vi "Running Average.vi"(8 "Error In":errorcluster, 11 "Async State Vars 2":T1) -> (0 "Error Out":errorcluster, 3 "Async State Vars out":T1)   [LabVIEW 2014, in "Waveform-Processing-Custom-Device Shared.lvlib" / "Running Average.lvlib"]
uses:
  Shared/Running Average/Running Average.lvlib
  Types/Async State Vars.ctl
  Types/Async FIFOs.ctl
  <vilib>/NI Veristand/Custom Device Waveform API/Single Waveform Read (DBL)/Single Waveform Read (DBL).lvclass
  <vilib>/NI Veristand/Custom Device Waveform API/Single Waveform Write (DBL)/Single Waveform Write (DBL).lvclass
  <vilib>/NI Veristand/Custom Device API/Waveform Data Reference.ctl
  <userlib>/Circular Buffer/Controls/Circular Buffer Operations.ctl
  <vilib>/Analysis/baseanly.llb/Mean (DBL).vi
  <userlib>/Circular Buffer/Instance VIs/Circular Buffer(2D DBL).vi
  <userlib>/Circular Buffer/Circular Buffer.lvlib
  <vilib>/Analysis/NI_AALBase.lvlib
  Waveform-Processing-Custom-Device Engine.lvlib
  <vilib>/NI Veristand/Custom Device API/Custom Device API.lvlib
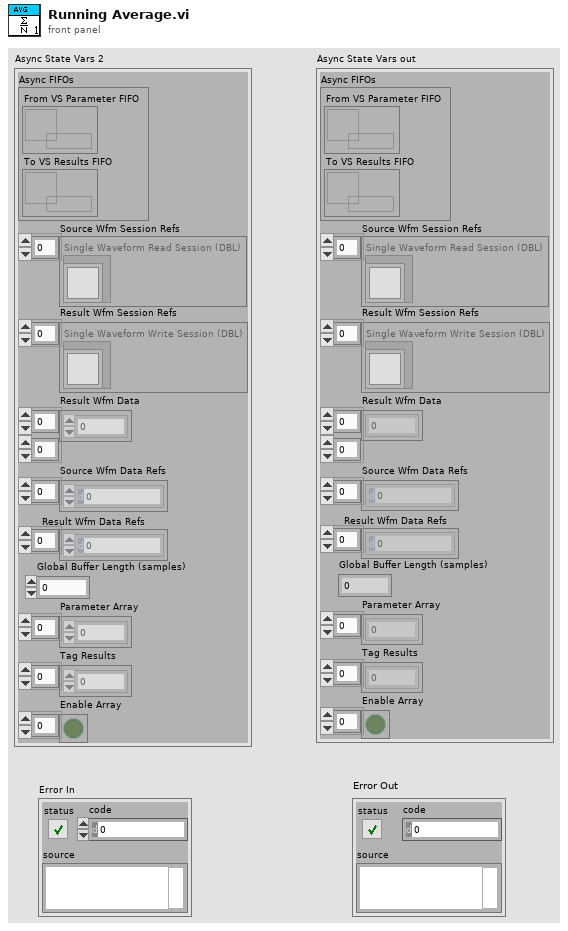
[diagram p1: front panel]
types:
  T1 = typedef "Waveform-Processing-Custom-Device Engine.lvlib/Async State Vars.ctl" = cluster{"Async FIFOs":T2, "Source Wfm Session Refs":refnum<class "Single Waveform Read (DBL).lvclass">[], "Result Wfm Session Refs":refnum<class "Single Waveform Write (DBL).lvclass">[], "Result Wfm Data":dbl[][], "Source Wfm Data Refs":T3[], "Result Wfm Data Refs":T3[], "Global Buffer Length (samples)":dbl, "Parameter Array":dbl[], "Tag Results":dbl[], "Enable Array":bool[]}
  T2 = typedef "Waveform-Processing-Custom-Device Engine.lvlib/Async FIFOs.ctl" = cluster{"From VS Parameter FIFO":refnum<k33>, "To VS Results FIFO":refnum<k33>}
  T3 = typedef "Custom Device API.lvlib/Waveform Data Reference.ctl" = i32
  T4 = typedef "Circular Buffer.lvlib/Circular Buffer Operations.ctl" = enum16{"Initialize", "Get Backlog", "Write", "Read (continuous)", "Read (most recent)"}
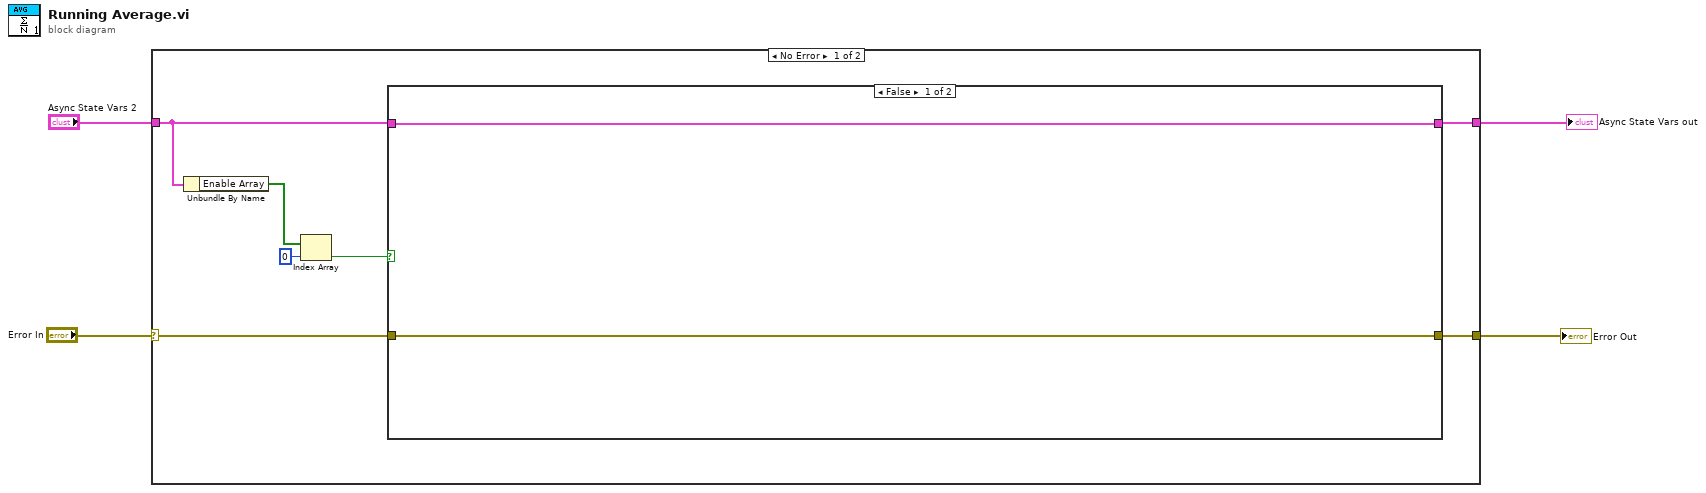
[diagram p0: block diagram]
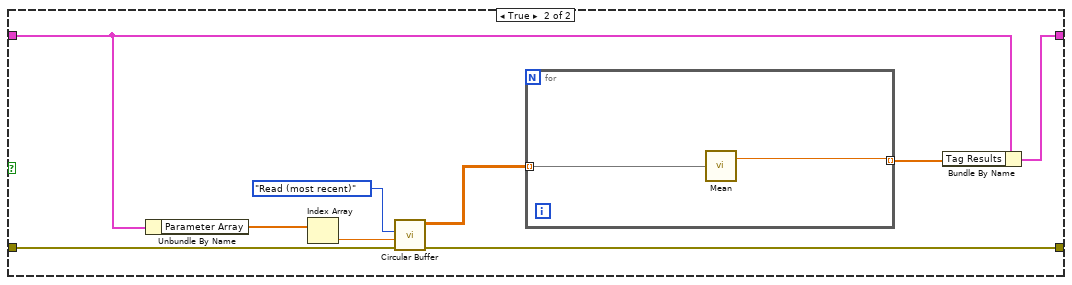
[diagram p2: hidden frame]
diagram:
  n1 = case shown="No Error" "Error In" {
    selector: "Error In" -> [w11 w26]
    tunnel: [w10 w26] -> w3
    tunnel: "Async State Vars 2" -> [w8 w25]
    tunnel: [w9 w25] -> w1
    frame No Error {
      n2 = Unbundle By Name(w8) -> ("Enable Array"=w7:bool[])
      n3 = Index Array(array=w7, index=0) -> (element=w6:bool)
      n4 = case shown="False" w6 {
        tunnel: w11 -> [w13 w20]
        tunnel: [w13 w19] -> w10
        tunnel: w8 -> [w12 w16]
        tunnel: [w12 w14] -> w9
        frame False {
        }
        frame True {
          n5 = Unbundle By Name(w16) -> ("Parameter Array"=w17:dbl[])
          n6 = Index Array(array=w17) -> (element=w18:dbl)  [unwired: 1 in]
          n7 = call-poly <userlib>:"Circular Buffer.vi"("error in (no error)"=w20, "Read Size"=w18, "Operation"=Circular_Buffer_Operations."Read (most recent)") -> ("error out"=w19:errorcluster, "Data Out"=w21:dbl[][])  [unwired: 5 in, 2 out]
          n8 = for {
            tunnel: w21 -> [w24] mode=indexing
            tunnel: [w23] -> w15 mode=indexing
            n9 = call-poly <vilib>:"Mean.vi"("X"=w24) -> ("mean"=w23:dbl)  [unwired: 1 out]
          }
          n10 = Bundle By Name(cluster=w16, "Tag Results"=w15) -> (w14:T1)
        }
      }
    }
    frame Error {
    }
  }
  "Error Out" <- w3
  "Async State Vars out" <- w1
